vi "Actor Teardown Decorator.vi"(10 "Error":errorcluster, 11 "Dev Actor in":refnum<class "Dev Actor.lvclass">) -> (0 "error out":errorcluster, 2 "Teardown?":bool, 3 "Dev Actor out":refnum<class "Dev Actor.lvclass">)   [LabVIEW 2021, in "Dev Actor.lvlib" / "Dev Actor.lvclass"]
uses:
  Dev Actor.lvclass
  Dev Actor.lvclass/Dev Actor.ctl
  src/LVCAM/LVCAM/Actor/Actor.lvclass
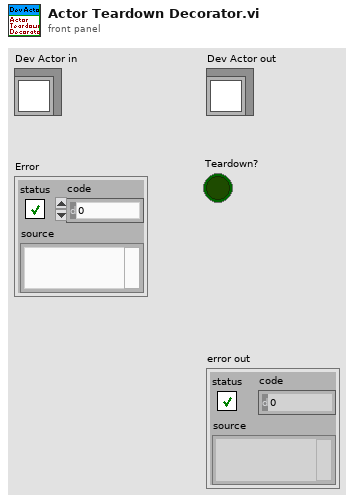
[diagram p1: front panel]
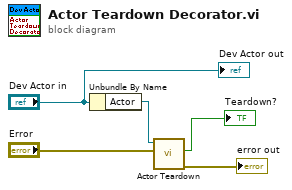
[diagram p0: block diagram]
diagram:
  n1 = Unbundle By Name("Dev Actor in") -> ("Actor"=w5:refnum<class "Actor.lvclass">)
  n2 = call-dynamic "Actor Teardown.vi"("Error"="Error", "Actor in"=w5) -> ("error out"=→"error out":errorcluster, "Teardown?"=→"Teardown?":bool)  [unwired: 7 in, 1 out]
  "Dev Actor out" <- "Dev Actor in"
